vi "RealTimeConversions.vi"() -> ()   [LabVIEW 2019]
uses:
  <vilib>/userDefined/High Color/IMAQdx.ctl
  <vilib>/vision/driver/NI_Vision_Acquisition_Software.lvlib
  RGB_To_Gray DLL Project/Project RGBToGray VI/RGBToGray.dll
  GrayToRGBAlternative DLL Project/VI Project/GrayToRGBAlternative.dll
panel:
  out "RGB Frame":T1(plugin-control)
  out "GrayScale Frame":T1(plugin-control)
  out "Array":dbl[](array[numeric])
  out "Elapsed time RGB in sec":dbl
  in  "stop":bool
  out "Camera Frame":T1(plugin-control)
  in  "Available Colormaps":T2
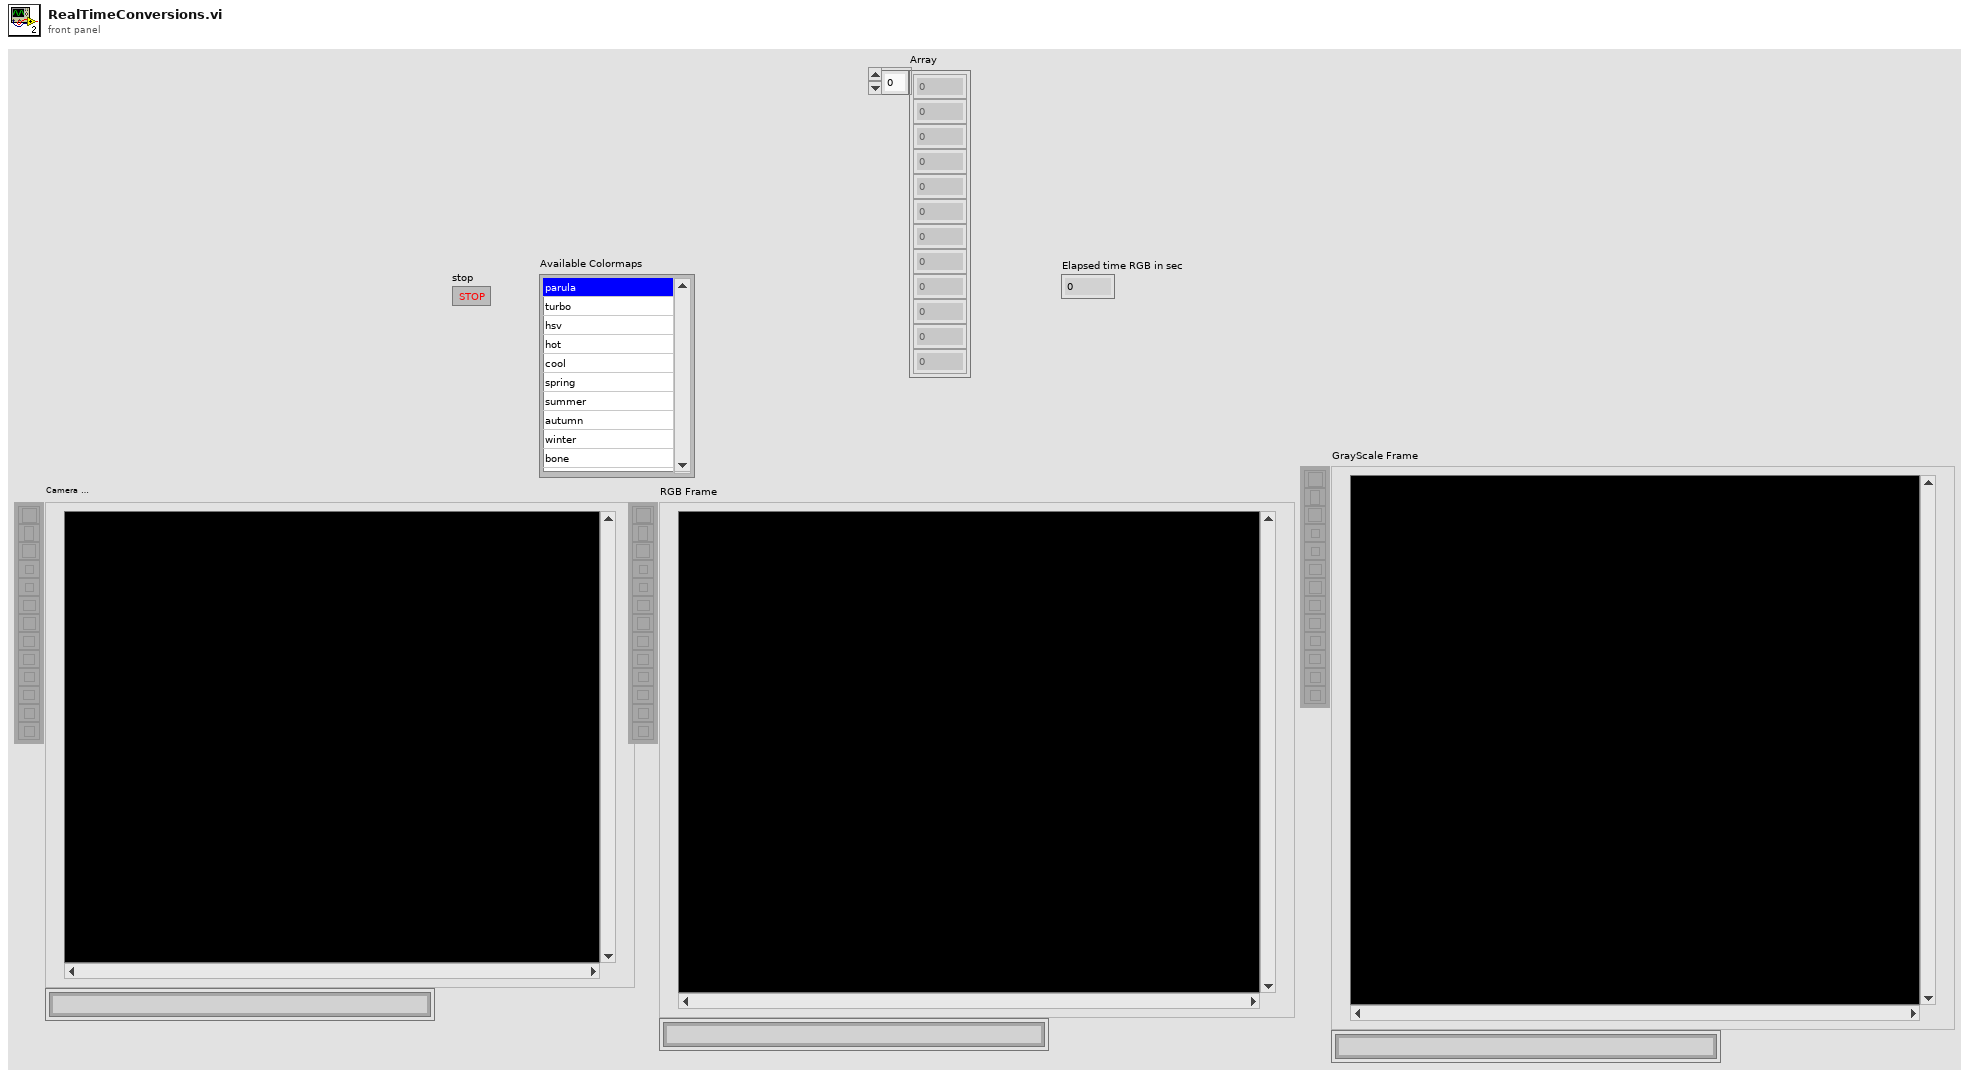
[diagram p1: front panel]
types:
  T1 = typedef "IMAQ Image.ctl" = refnum<image>
  T2 = typedef "Control 1.ctl" = i32
  T3 = typedef "Image Type" = u32
  T4 = typedef "IMAQdx.ctl" = refnum<k21>
  T5 = enum32{"Map Pixel Pointer", "Unmap Pixel Pointer", "Get Pixels Infos"}
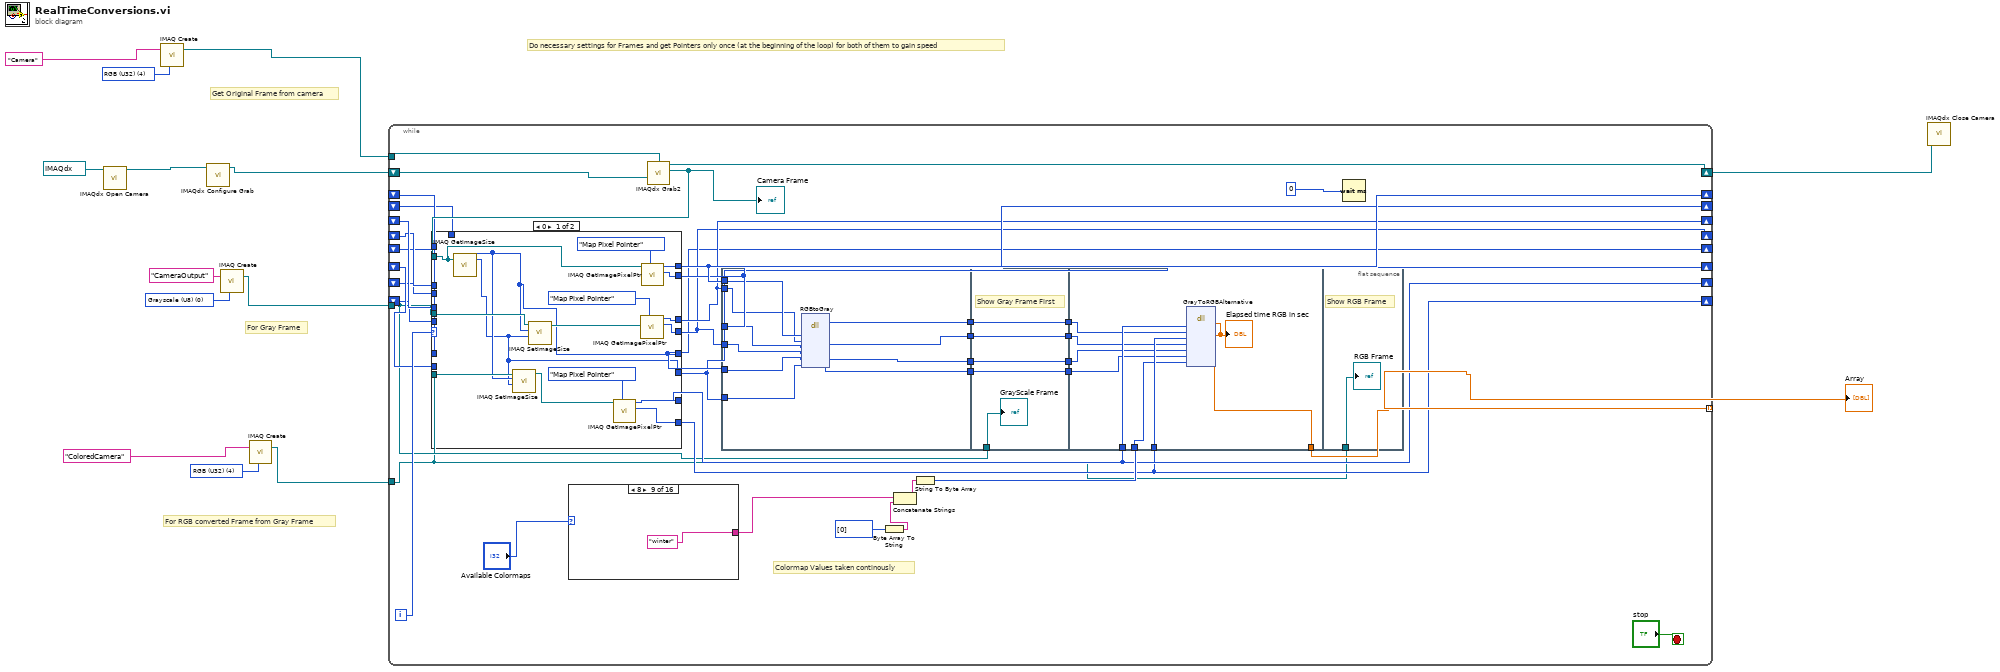
[diagram p0: block diagram]
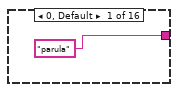
[diagram p3: hidden frame]
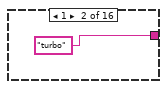
[diagram p4: hidden frame]
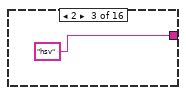
[diagram p5: hidden frame]
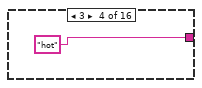
[diagram p6: hidden frame]
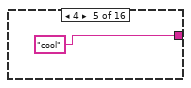
[diagram p7: hidden frame]
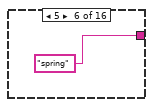
[diagram p8: hidden frame]
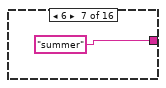
[diagram p9: hidden frame]
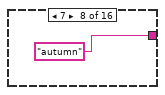
[diagram p10: hidden frame]
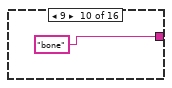
[diagram p11: hidden frame]
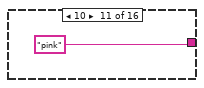
[diagram p12: hidden frame]
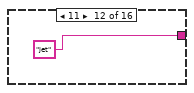
[diagram p13: hidden frame]
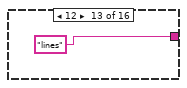
[diagram p14: hidden frame]
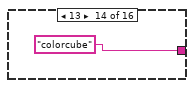
[diagram p15: hidden frame]
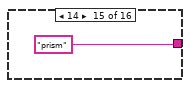
[diagram p16: hidden frame]
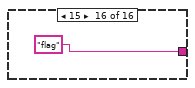
[diagram p17: hidden frame]
diagram:
  w6 = T3 4 items=["Grayscale (U8)", "Grayscale (I16)", "Grayscale (SGL)", "Complex (CSG)", "RGB (U32)", "HSL (U32)", "RGB (U64)", "Grayscale (U16)"] ("Image Type")
  w9 = T3 0 items=["Grayscale (U8)", "Grayscale (I16)", "Grayscale (SGL)", "Complex (CSG)", "RGB (U32)", "HSL (U32)", "RGB (U64)", "Grayscale (U16)"] ("Image Type")
  w11 = T3 4 items=["Grayscale (U8)", "Grayscale (I16)", "Grayscale (SGL)", "Complex (CSG)", "RGB (U32)", "HSL (U32)", "RGB (U64)", "Grayscale (U16)"] ("Image Type")
  # "Do necessary settings for Frames and get Pointers only once (at the beginning of the loop) for both of them to gain speed"
  # "For RGB converted Frame from Gray Frame"
  # "For Gray Frame"
  # "Get Original Frame from camera"
  n1 = call <vilib>:"IMAQdx Open Camera.vi"("Session In"=T4 "cam0") -> ("Session Out"=w13:T4)  [unwired: 9 in, 1 out]
  n2 = call "IMAQ Create"("Image Name"="Camera", "Image Type"=w11) -> ("New Image"=w4:T1)  [unwired: 3 in, 1 out]
  n3 = call <vilib>:"IMAQdx Configure Grab.vi"("Session In"=w13) -> ("Session Out"=w5:T4)  [unwired: 9 in, 1 out]
  n4 = call "IMAQ Create"("Image Name"="CameraOutput", "Image Type"=w9) -> ("New Image"=w2:T1)  [unwired: 3 in, 1 out]
  n5 = call "IMAQ Create"("Image Name"="ColoredCamera", "Image Type"=w6) -> ("New Image"=w3:T1)  [unwired: 3 in, 1 out]
  n6 = while {
    shift-right: [w52] -> w8
    shift-left: w5 -> [w54]
    tunnel: w3 -> [w15]
    tunnel: w4 -> [w44]
    tunnel: w2 -> [w17]
    shift-right: [w41] -> _
    shift-left: _ -> [w39]
    shift-right: [w40] -> _
    shift-left: _ -> [w38]
    shift-right: [w37] -> _
    shift-left: _ -> [w36]
    shift-right: [w35] -> _
    shift-left: _ -> [w34]
    shift-right: [w33] -> _
    shift-left: _ -> [w32]
    shift-right: [w31] -> _
    shift-left: _ -> [w30]
    shift-right: [w29] -> _
    shift-left: _ -> [w28]
    shift-right: [w27] -> _
    shift-left: _ -> [w26]
    tunnel: [w16] -> w1 mode=indexing
    i -> [w43]
    stop <- "stop" stop-if-true
    # "Colormap Values taken continously"
    n7 = case shown="8" "Available Colormaps" {
      tunnel: ["parula" "turbo" "hsv" "hot" "cool" "spring" "summer" "autumn" "winter" "bone" "pink" "jet" "lines" "colorcube" "prism" "flag"] -> w46
      frame 0, Default {
      }
      frame 1 {
      }
      frame 2 {
      }
      frame 3 {
      }
      frame 4 {
      }
      frame 5 {
      }
      frame 6 {
      }
      frame 7 {
      }
      frame 8 {
      }
      frame 9 {
      }
      frame 10 {
      }
      frame 11 {
      }
      frame 12 {
      }
      frame 13 {
      }
      frame 14 {
      }
      frame 15 {
      }
    }
    n8 = call <vilib>:"IMAQdx Grab2.vi"("Image In"=w44, "Session In"=w54) -> ("Image Out"=w42:T1, "Session Out"=w52:T4)  [unwired: 6 in, 2 out]
    "Camera Frame" <- w42
    n9 = case shown="0" w43 {
      tunnel: w42 -> [w59 _]
      tunnel: w17 -> [w65 _]
      tunnel: w15 -> [w64 _]
      tunnel: [w63 w72] -> w29
      tunnel: [w62 w71] -> w27
      tunnel: [w61 w76] -> w37
      tunnel: [w60 w75] -> w35
      tunnel: [w58 w74] -> w33
      tunnel: [w57 w73] -> w31
      tunnel: [w56 w78] -> w41
      tunnel: [w55 w77] -> w40
      tunnel: w39 -> [_ w78]
      tunnel: w38 -> [_ w77]
      tunnel: w36 -> [_ w76]
      tunnel: w34 -> [_ w75]
      tunnel: w32 -> [_ w74]
      tunnel: w30 -> [_ w73]
      tunnel: w28 -> [_ w72]
      tunnel: w26 -> [_ w71]
      frame 0 {
        n10 = call "IMAQ GetImageSize"("Image"=w59) -> ("Y Resolution"=w57:i32, "X Resolution"=w58:i32)  [unwired: 3 in, 1 out]
        n11 = call "IMAQ SetImageSize"("Y Resolution"=w57, "X Resolution"=w58, "Image"=w64) -> ("Image Out"=w68:T1)  [unwired: 2 in, 1 out]
        n12 = call "IMAQ SetImageSize"("Y Resolution"=w57, "X Resolution"=w58, "Image"=w65) -> ("Image Out"=w66:T1)  [unwired: 2 in, 1 out]
        n13 = call "IMAQ GetImagePixelPtr"("Function"=T5."Map Pixel Pointer", "Image"=w68) -> ("LineWidth(Pixels)"=w62:i32, "Pixel Pointer out"=w63:u64)  [unwired: 4 in, 4 out]
        n14 = call "IMAQ GetImagePixelPtr"("Function"=T5."Map Pixel Pointer", "Image"=w66) -> ("LineWidth(Pixels)"=w60:i32, "Pixel Pointer out"=w61:u64)  [unwired: 4 in, 4 out]
        n15 = call "IMAQ GetImagePixelPtr"("Function"=T5."Map Pixel Pointer", "Image"=w59) -> ("LineWidth(Pixels)"=w55:i32, "Pixel Pointer out"=w56:u64)  [unwired: 4 in, 4 out]
      }
      frame 1, Default {
      }
    }
    n16 = flat-sequence {
      tunnel: [w104] -> w25
      tunnel: [w103] -> w23
      tunnel: [w102] -> w21
      tunnel: [w101] -> w19
      tunnel: w41 -> [w100]
      tunnel: w37 -> [w99]
      tunnel: w40 -> [w98]
      tunnel: w35 -> [w97]
      tunnel: w33 -> [w96]
      tunnel: w31 -> [w95]
      tunnel: w25 -> [w109]
      tunnel: [w109] -> w24
      tunnel: w23 -> [w108]
      tunnel: [w108] -> w22
      tunnel: w21 -> [w107]
      tunnel: [w107] -> w20
      tunnel: w19 -> [w106]
      tunnel: [w106] -> w18
      tunnel: w17 -> [w105]
      tunnel: w45 -> [w111]
      tunnel: w24 -> [w116]
      tunnel: w22 -> [w114]
      tunnel: w20 -> [w113]
      tunnel: w18 -> [w112]
      tunnel: w29 -> [w117]
      tunnel: w27 -> [w115]
      tunnel: [w110] -> w16
      tunnel: w15 -> [w118]
      frame #0 {
        n17 = dll-call lib="C:/Users/byald/Desktop/EE-433 Project Group1/RGB_To_Gray DLL Project/Project RGBToGray VI/RGBToGray.dll" fn="RGBtoGray"("RGBImage"=w100, "GrayImage"=w99, "LVLineWidthRGB"=w98, "LVLineWidthGray"=w97, "LVWidth"=w96, "LVHeight"=w95) -> ("GrayImage"=w104:u64, "LVLineWidthGray"=w103:i32, "LVWidth"=w102:i32, "LVHeight"=w101:i32)  [unwired: 6 in, 2 out]
      }
      frame #1 {
        # "Show Gray Frame First"
        "GrayScale Frame" <- w105
      }
      frame #2 {
        n18 = dll-call lib="C:/Users/byald/Desktop/EE-433 Project Group1/GrayToRGBAlternative DLL Project/VI Project/GrayToRGBAlternative.dll" fn="GrayToRGBAlternative"("RGBImage"=w117, "GrayImage"=w116, "LVLineWidthRGB"=w115, "LVLineWidthGray"=w114, "LVWidth"=w113, "LVHeight"=w112, "ColorMap"=w111) -> ("return type"=w110:dbl)  [unwired: 10 in, 2 out]
        "Elapsed time RGB in sec" <- w110
      }
      frame #3 {
        # "Show RGB Frame"
        "RGB Frame" <- w118
      }
    }
    n19 = Byte Array To String(unsigned byte array=u8[] [0]) -> (string=w48:string)
    n20 = Concatenate Strings(w46, w48) -> (w47:string)
    n21 = String To Byte Array(string=w47) -> (unsigned byte array=w45:u8[])
    n22 = Wait (ms)(milliseconds to wait=u32 0) -> ()  [unwired: 1 out]
  }
  "Array" <- w1
  n23 = call <vilib>:"IMAQdx Close Camera.vi"("Session In"=w8) -> ()  [unwired: 10 in, 1 out]
